vi "parse websocket length header.vi"(11 "header string":string) -> (2 "length":u8, 3 "first byte":T1 {"opcode" format="%.0x"})   [LabVIEW 2016, in "websocket upgrade handler.lvclass"]
uses:
  websocket upgrade handler.lvclass
  first byte header.ctl
  opcode.ctl
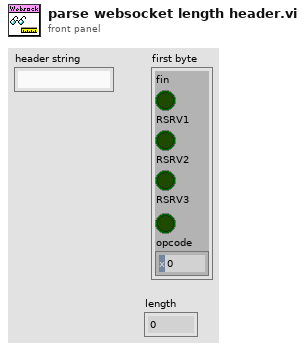
[diagram p1: front panel]
types:
  T1 = typedef "websocket upgrade handler.lvclass/first byte header.ctl" = cluster{"fin":bool, "RSRV1":bool, "RSRV2":bool, "RSRV3":bool, "opcode":u8}
  T2 = typedef "websocket upgrade handler.lvclass/opcode.ctl" = u8
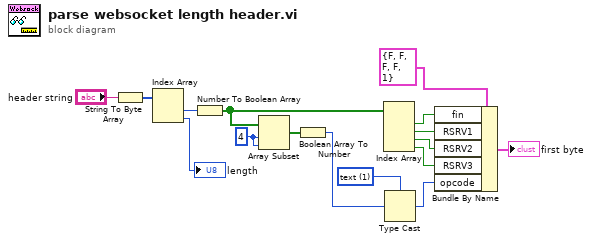
[diagram p0: block diagram]
diagram:
  w9 = T2 1 items=["continuation"=0, "text"=1, "binary"=2, "close"=8, "ping"=9, "pong"=10] ("opcode")
  w6 = 4 ("index")
  n1 = String To Byte Array(string="header string") -> (unsigned byte array=w2:u8[])
  n2 = Index Array(array=w2) -> (element #1=w4:u8, element #2=→"length":u8)  [unwired: 2 in]
  n3 = Number To Boolean Array(number=w4) -> (Boolean array=w5:bool[])
  n4 = Array Subset(array=w5, index=w6, length=w6) -> (w7:bool[])
  n5 = Boolean Array To Number(Boolean array=w7) -> (number=w8:u32)
  n6 = Index Array(array=w5) -> (element #1=w11:bool, element #2=w15:bool, element #3=w14:bool, element #4=w13:bool)  [unwired: 4 in]
  n7 = Type Cast(type=w9, x=w8) -> (*(type *) &x=w12:T2)
  n8 = Bundle By Name(cluster=T1 {"fin"=FALSE, "RSRV1"=FALSE, "RSRV2"=FALSE, "RSRV3"=FALSE, "opcode"=1} ("first byte"), "fin"=w11, "RSRV1"=w15, "RSRV2"=w14, "RSRV3"=w13, "opcode"=w12) -> (→"first byte":T1)
